vi "Supported Smart Syntax Representation.vi"(0 "Message Popup in":refnum<class "Array Functions.lvclass">, 11 "error in (no error)":errorcluster) -> (4 "Message Popup out":refnum<class "Array Functions.lvclass">, 6 "Smart Syntax Representation List":string[](array[string]), 15 "error out":errorcluster)   [LabVIEW 2019, in "Array Functions.lvclass"]
uses:
  Array Functions.lvclass
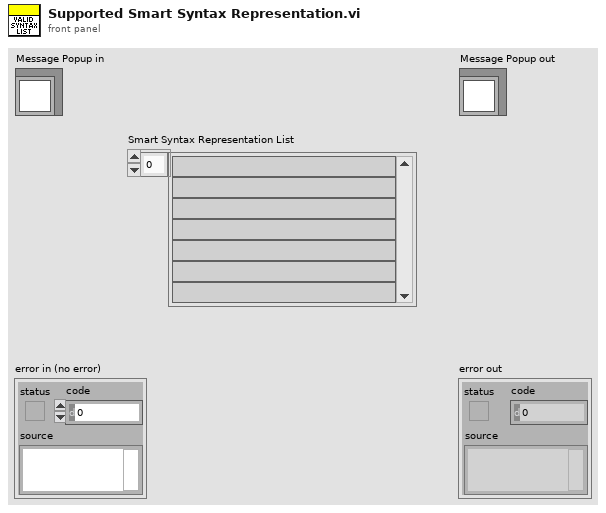
[diagram p1: front panel]
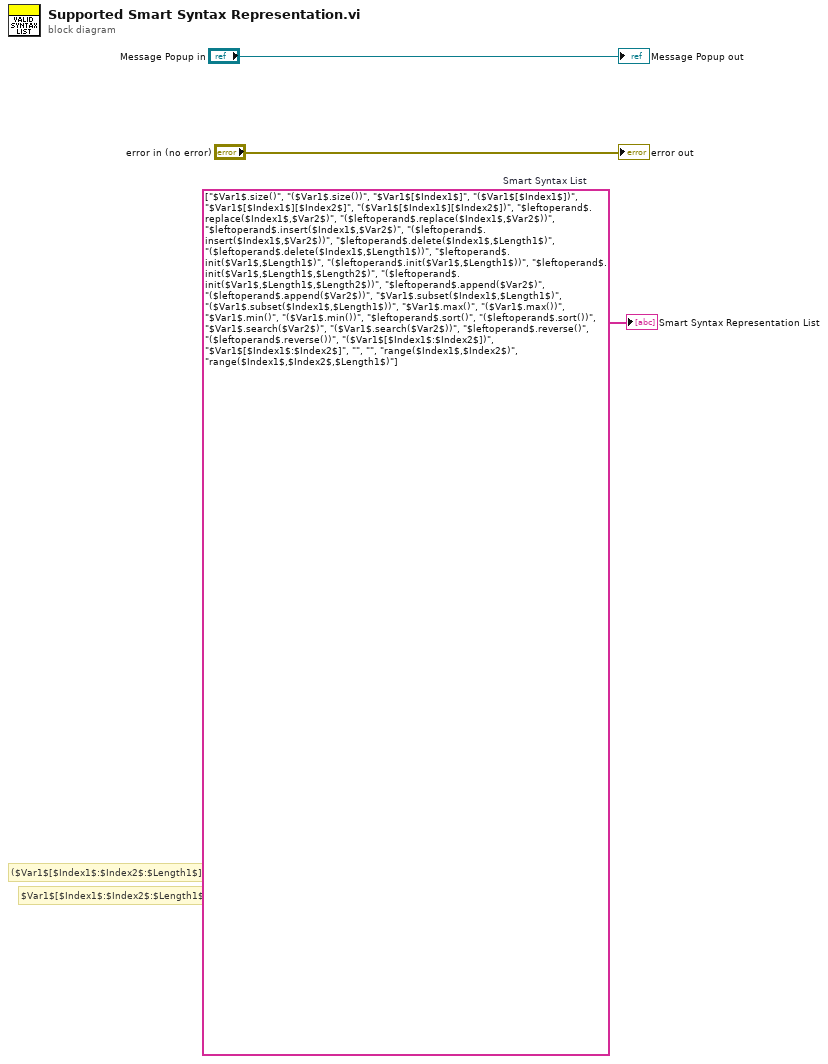
[diagram p0: block diagram]
diagram:
  w1 = string[] ["$Var1$.size()", "($Var1$.size())", "$Var1$[$Index1$]", "($Var1$[$Index1$])", "$Var1$[$Index1$][$Index2$]", "($Var1$[$Index1$][$Index2$])", "$leftoperand$.replace($Index1$,$Var2$)", "($leftoperand$.replace($Index1$,$Var2$))", "$leftoperand$.insert($Index1$,$Var2$)", "($leftoperand$.insert($Index1$,$Var2$))", "$leftoperand$.delete($Index1$,$Length1$)", "($leftoperand$.delete($Index1$,$Length1$))", "$leftoperand$.init($Var1$,$Length1$)", "($leftoperand$.init($Var1$,$Length1$))", "$leftoperand$.init($Var1$,$Length1$,$Length2$)", "($leftoperand$.init($Var1$,$Length1$,$Length2$))", "$leftoperand$.append($Var2$)", "($leftoperand$.append($Var2$))", "$Var1$.subset($Index1$,$Length1$)", "($Var1$.subset($Index1$,$Length1$))", "$Var1$.max()", "($Var1$.max())", "$Var1$.min()", "($Var1$.min())", "$leftoperand$.sort()", "($leftoperand$.sort())", "$Var1$.search($Var2$)", "($Var1$.search($Var2$))", "$leftoperand$.reverse()", "($leftoperand$.reverse())", "($Var1$[$Index1$:$Index2$])", "$Var1$[$Index1$:$Index2$]", "", "", "range($Index1$,$Index2$)", "range($Index1$,$Index2$,$Length1$)"]  # Smart Syntax List
  # "($Var1$[$Index1$:$Index2$:$Length1$])"
  # "$Var1$[$Index1$:$Index2$:$Length1$]"
  "error out" <- "error in (no error)"
  "Message Popup out" <- "Message Popup in"
  "Smart Syntax Representation List" <- w1
